vi "Copy .LLB to NI VeriStand dir.vi"(5 "Files Generated by Build":path[](array[path]), 6 "Top Level/Always Included VIs":path[](array[path]), 7 "Destination Path":path, 8 "error in (no error)":errorcluster, 9 "Target Name":string, 10 "Build Specification Name":string, 11 "Project Path":path) -> (0 "error out":errorcluster)   [LabVIEW 2019]
doc: "This VI is called after each run of a build specification. The VI will copy the generated LLB (Engine or System Explorer) into the VeriStand Custom Device folder (...\\Documents\\National Instruments\\NI VeriStand 2013...)."
uses:
  <vilib>/Utility/sysdir.llb/System Directory Type.ctl
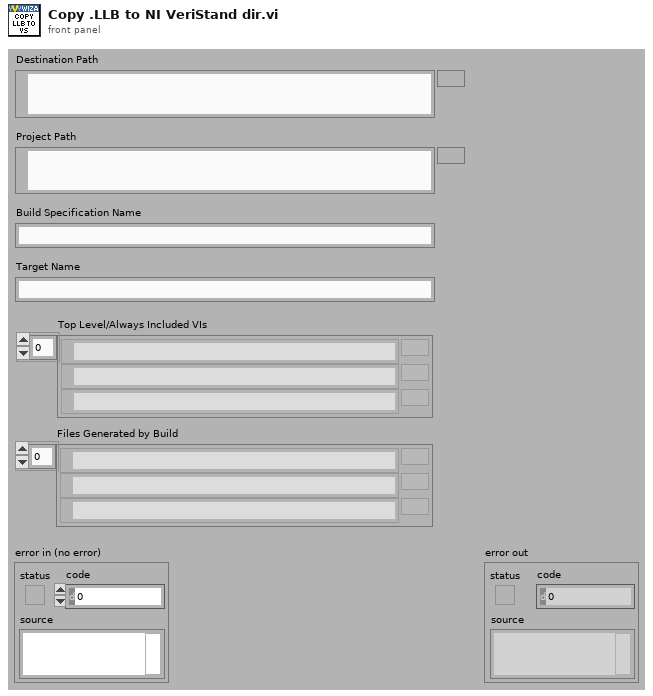
[diagram p1: front panel]
types:
  T1 = typedef "System Directory Type.ctl" = i32
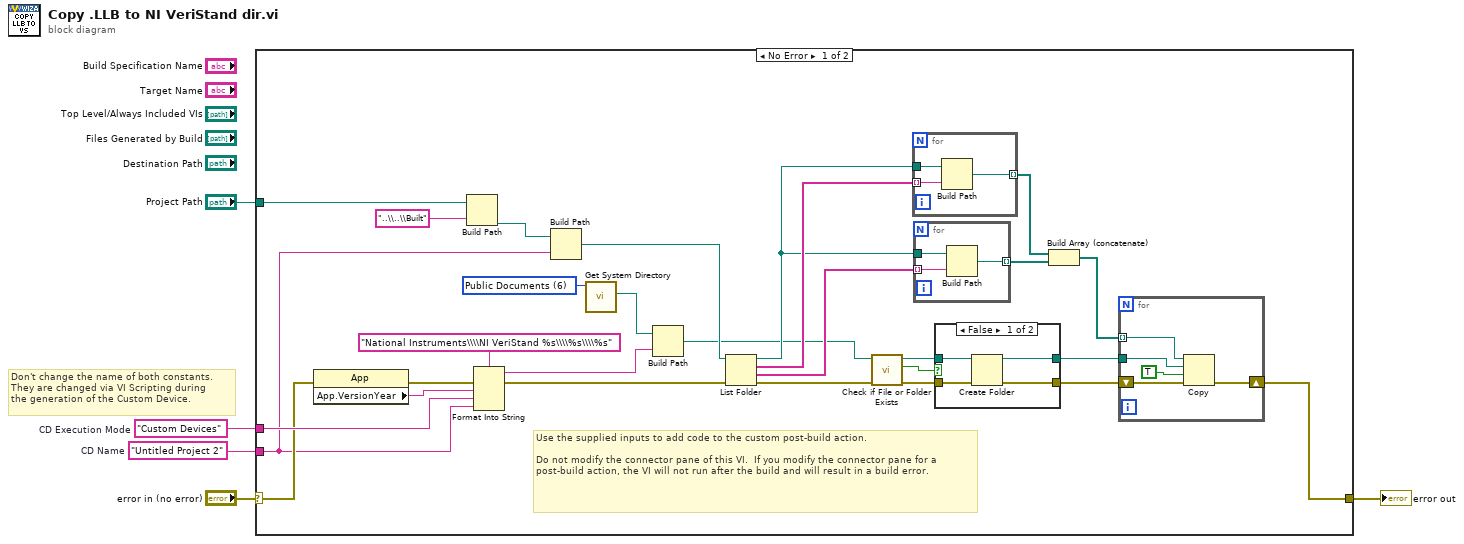
[diagram p0: block diagram]
diagram:
  w2 = "Untitled Project 2"  # CD Name
  w3 = "Custom Devices"  # CD Execution Mode
  # "Don't change the name of both constants.\nThey are changed via VI Scripting during\nthe generation of the Custom Device."
  n1 = case shown="No Error" "error in (no error)" {
    selector: "error in (no error)" -> [w12 w51]
    tunnel: [w15 w51] -> w1
    tunnel: "Project Path" -> [w8 _]
    tunnel: w3 -> [w13 _]
    tunnel: w2 -> [w10 _]
    frame No Error {
      w19 = T1 6 items=["User Home"=0, "User Desktop"=1, "User Documents"=2, "User Application Data"=3, "User Preferences"=4, "User Temporary"=5, "Public Documents"=6, "Public Application Data"=7, "Public Preferences"=8, "Public Cache"=13, "System Core Libraries"=9, "System Installed Libraries"=10, "Application Files"=11, "Boot Volume Root"=12] ("system directory type")
      # "Use the supplied inputs to add code to the custom post-build action.\n\nDo not modify the connector pane of this VI.  If you modify the connector pane for a post-build action, the VI will not run after the build and will result in a build error."
      n2 = property class="App"(error in=w12) -> (error out=w18:errorcluster, "App.VersionYear"=w17:string)  [unwired: 1 in, 1 out]
      n3 = Build Path(base path=w8, name or relative path="..\\..\\Built") -> (appended path=w22:path)
      n4 = Format Into String(format string="National Instruments\\\\NI VeriStand %s\\\\%s\\\\%s" ("name or relative path"), error in=w18, w17, w13, w10) -> (resulting string=w21:string, error out=w11:errorcluster)  [unwired: 1 in]
      n5 = Build Path(base path=w22, name or relative path=w10) -> (appended path=w24:path)
      n6 = call <vilib>:"Get System Directory.vi"("system directory type"=w19) -> ("system directory"=w20:path)  [unwired: 10 in]
      n7 = Build Path(base path=w20, name or relative path=w21) -> (appended path=w14:path)
      n8 = List Folder(path=w24, error in=w11) -> (path out=w26:path, filenames=w33:string[], folder names=w27:string[], error out=w23:errorcluster)  [unwired: 2 in]
      n9 = call <vilib>:"Check if File or Folder Exists.vi"("error in (no error)"=w23, "path"=w14) -> ("error out"=w28:errorcluster, "file or folder exists?"=w30:bool, "dup path"=w29:path)  [unwired: 7 in]
      n10 = for {
        tunnel: w33 -> [w49] mode=indexing
        tunnel: w26 -> [w50]
        tunnel: [w48] -> w32 mode=indexing
        n11 = Build Path(base path=w50, name or relative path=w49) -> (appended path=w48:path)
      }
      n12 = for {
        tunnel: w27 -> [w46] mode=indexing
        tunnel: w26 -> [w47]
        tunnel: [w45] -> w25 mode=indexing
        n13 = Build Path(base path=w47, name or relative path=w46) -> (appended path=w45:path)
      }
      n14 = case shown="False" w30 {
        tunnel: w29 -> [w37 w39]
        tunnel: w28 -> [w36 w38]
        tunnel: [w35 w39] -> w7
        tunnel: [w34 w38] -> w6
        frame False {
          n15 = Create Folder(path (use dialog)=w37, error in=w36) -> (created path=w35:path, error out=w34:errorcluster)  [unwired: 1 in, 1 out]
        }
        frame True {
        }
      }
      n16 = Build Array (concatenate)(w32, w25) -> (w31:path[])
      n17 = for {
        tunnel: w31 -> [w41] mode=indexing
        shift-right: [w42] -> w15
        shift-left: w6 -> [w43]
        tunnel: w7 -> [w40]
        n18 = Copy(8:w43, 9:TRUE ("overwrite (F)"), 10:w40, 11:w41) -> (0:w42:errorcluster)  [unwired: 1 in, 2 out]
      }
    }
    frame Error {
    }
  }
  "error out" <- w1
